vi "Send Raw Command.vi"(8 "error in":errorcluster, 10 "Raw Command":u8[](array[numeric]), 11 "ProXR_IO in":refnum<class "ProXR.lvclass">) -> (0 "error out":errorcluster, 3 "ProXR_IO out":refnum<class "ProXR.lvclass">)   [LabVIEW 2019, in "ProXR.lvlib" / "ProXR.lvclass"]
uses:
  Library/ProXR.lvclass
  Library/ProXR.lvclass/ProXR.ctl
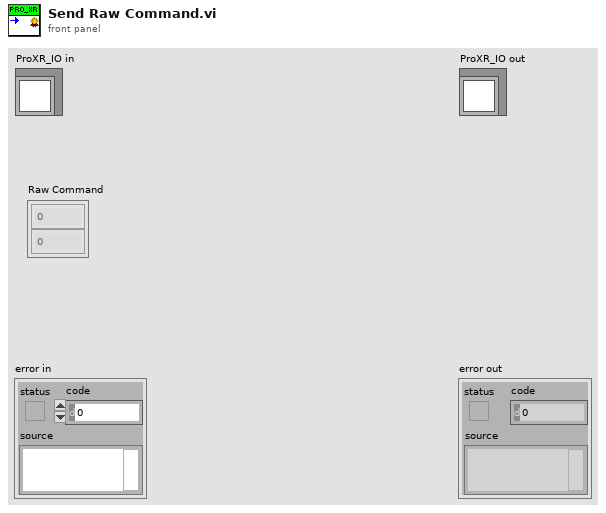
[diagram p1: front panel]
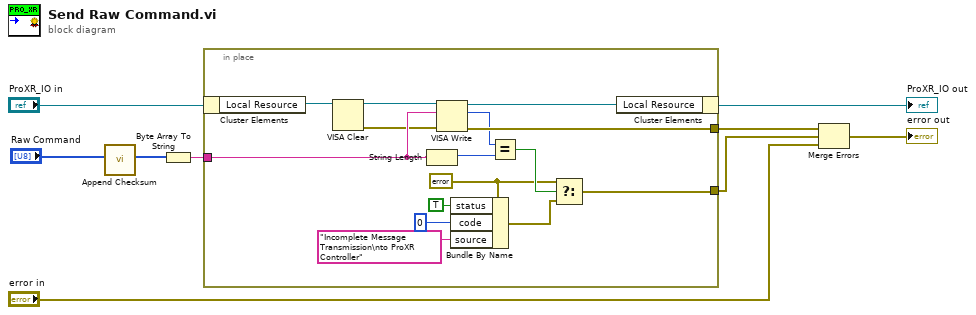
[diagram p0: block diagram]
diagram:
  n1 = call "Append Checksum.vi"("Message"="Raw Command") -> ("Message w cksum"=w1:u8[])  [unwired: 9 in, 1 out]
  n2 = Byte Array To String(unsigned byte array=w1) -> (string=w6:string)
  n3 = in-place {
    in-place-border: [w23] -> w7
    in-place-border: w6 -> [w22]
    in-place-border: [w16] -> w5
    w17 = errorcluster {"status"=FALSE, "code"=0, "source"=""} ("error in")
    n4 = in-place-cluster #1("ProXR_IO in") -> ("Local Resource"=w12:refnum<visa-resource-name>)
    n5 = VISA Clear(VISA resource name=w12) -> (VISA resource name out=w11:refnum<visa-resource-name>, error out=w10:errorcluster)  [unwired: 1 in]
    n6 = String Length(string=w22) -> (length=w20:i32)
    n7 = VISA Write(VISA resource name=w11, write buffer=w22, error in (no error)=w10) -> (VISA resource name out=w24:refnum<visa-resource-name>, return count=w21:u32, error out=w23:errorcluster)
    n8 = Bundle By Name(cluster=w17, "status"=TRUE, "code"=0, "source"="Incomplete Message Transmission\nto ProXR Controller") -> (w13:errorcluster)
    n9 = Equal?(x=w21, y=w20) -> (x = y?=w18:bool)
    n10 = Select(t=w17, s=w18, f=w13) -> (s? t:f=w16:errorcluster)
    n11 = in-place-cluster #1("Local Resource"=w24) -> (→"ProXR_IO out":refnum<class "ProXR.lvclass">)
  }
  n12 = Merge Errors(w7, w5, "error in") -> (→"error out":errorcluster)
